vi "script_split_command.vi"(1 "Full command":string) -> (0 "Argv":string[](array[string]))   [LabVIEW 2015]
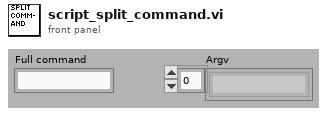
[diagram p1: front panel]
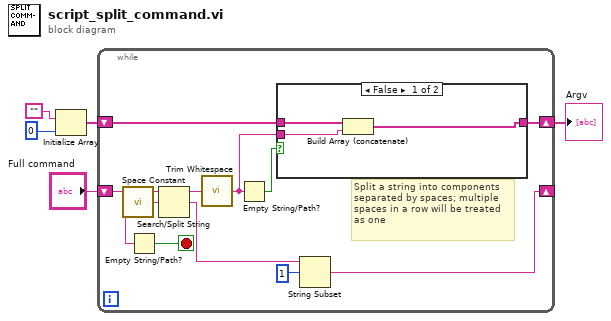
[diagram p0: block diagram]
diagram:
  n1 = Initialize Array("", 0 ("dimension size")) -> (w4:string[])
  n2 = while {
    shift-right: [w7] -> _
    shift-left: "Full command" -> [w10]
    shift-right: [w11] -> w5
    shift-left: w4 -> [w13]
    stop <- w9 stop-if-true
    # "Split a string into components\nseparated by spaces; multiple\nspaces in a row will be treated\nas one"
    n3 = call <vilib>:"Space Constant.vi"() -> ("String"=w16:string)
    n4 = Empty String/Path?(string/path=w10) -> (empty?=w9:bool)
    n5 = Search/Split String(string=w10, search string/char (-)=w16) -> (substring before match=w15:string, match + rest of string=w8:string)  [unwired: 1 in, 1 out]
    n6 = call <vilib>:"Trim Whitespace.vi"("string"=w15) -> ("trimmed string"=w12:string)  [unwired: 1 in]
    n7 = Empty String/Path?(string/path=w12) -> (empty?=w14:bool)
    n8 = case shown="False" w14 {
      tunnel: w13 -> [w19 w20]
      tunnel: w12 -> [w18 _]
      tunnel: [w17 w20] -> w11
      frame False {
        n9 = Build Array (concatenate)(w19, w18) -> (w17:string[])
      }
      frame True {
      }
    }
    n10 = String Subset(string=w8, offset (0)=1) -> (substring=w7:string)  [unwired: 1 in]
  }
  "Argv" <- w5
